vi "U2722A_Source_V_Measure_I_Ver.1.0.vi"(8 "error in (no error)":errorcluster, 9 "Output Level (1.0 V)":dbl=1.0, 10 "Channel (1: Channel 1)":u16(ring)=1 items=["Channel 1"=1, "Channel 2"=2, "Channel 3"=3], 11 "VISA resource name":refnum<visa-resource-name>) -> (0 "error out":errorcluster, 1 "Actual Current Level (A)":dbl format="%.2g", 3 "VISA resource name out":refnum<visa-resource-name>)   [LabVIEW 2018]
doc: "Configures the channel to output in source voltage mode."
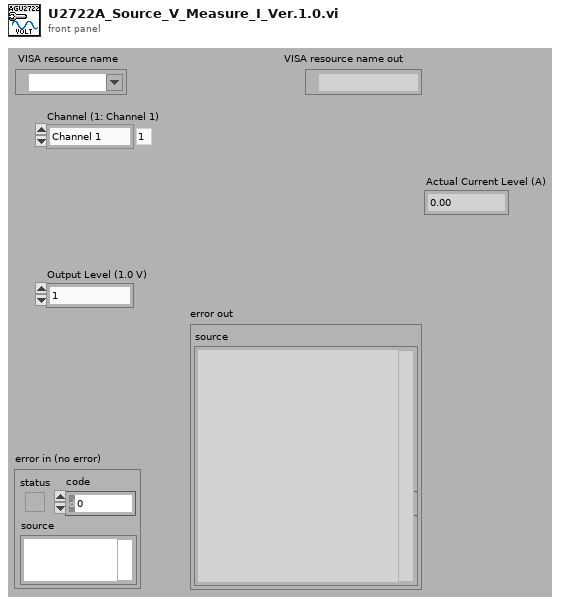
[diagram p1: front panel]
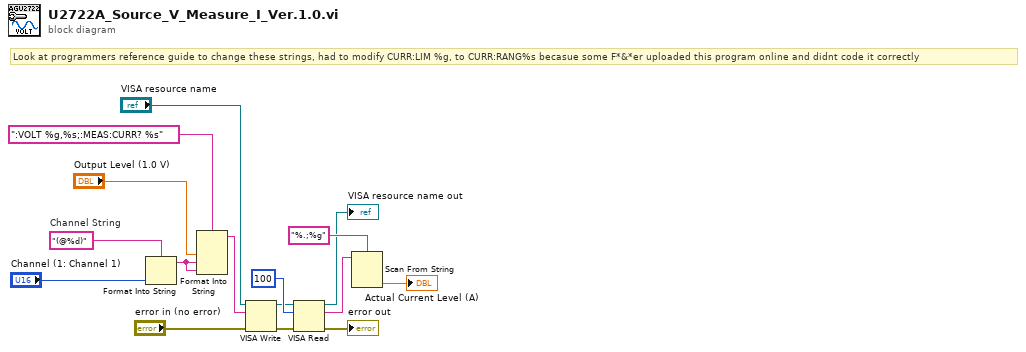
[diagram p0: block diagram]
diagram:
  w13 = "(@%d)"  # Channel String
  # "Look at programmers reference guide to change these strings, had to modify CURR:LIM %g, to CURR:RANG%s becasue some F*&*er uploaded this program online and didnt code it correctly"
  n1 = Format Into String(format string=w13, "Channel (1: Channel 1)") -> (resulting string=w5:string)  [unwired: 2 in, 1 out]
  n2 = Format Into String(format string=":VOLT %g,%s;:MEAS:CURR? %s", "Output Level (1.0 V)", w5, w5) -> (resulting string=w12:string)  [unwired: 2 in, 1 out]
  n3 = VISA Write(VISA resource name="VISA resource name", write buffer=w12, error in (no error)="error in (no error)") -> (VISA resource name out=w4:refnum<visa-resource-name>, error out=w3:errorcluster)  [unwired: 1 out]
  n4 = VISA Read(VISA resource name=w4, byte count=u32 100, error in (no error)=w3) -> (VISA resource name out=→"VISA resource name out":refnum<visa-resource-name>, read buffer=w8:string, error out=→"error out":errorcluster)  [unwired: 1 out]
  n5 = Scan From String(format string="%.;%g", input string=w8) -> (output 1=→"Actual Current Level (A)":dbl)  [unwired: 3 in, 3 out]
